vi "SPCC_Assignment_Simulation.vi"() -> ()   [LabVIEW 2023]
uses:
  e3bf969a-aac0-434e-a3ae-6fd923815a2a.vi
  48b219de-f1ff-457e-af6a-4fba154d072f.vi
  41e50873-912a-4f0f-ad4e-86c641a04fe7.vi
  6f4b4a78-1284-474b-8f97-6c78d8e6e227.vi
  13f19a0c-8ff0-4895-a446-3eb92896fe58.vi
  ebdab617-ba7c-440d-b82c-f0f3d50a62cd.vi
  86e3c8e6-2093-4571-a988-bd0a6019ca9d.vi
  4dc1e517-941c-447c-bbf6-cb1460c6f39a.vi
  a41b0926-84b4-47fe-bcd1-4c6ccf125de5.vi
  03f30388-958a-4886-846a-0cab3cf4eed9.vi
  04fb8fff-2e92-42f1-ae9c-eeda405f3134.vi
  4105182e-33e6-4150-80c3-b8c49d90c377.vi
panel:
  in  "btnStop":bool
  in  "A1":bool
  in  "A6":bool
  in  "A5":bool
  in  "A4":bool
  in  "A3":bool
  in  "A2":bool
  in  "B1":bool
  in  "B6":bool
  in  "B5":bool
  in  "B4":bool
  in  "B3":bool
  in  "B2":bool
  in  "T1":bool
  in  "T6":bool
  in  "T5":bool
  in  "T4":bool
  in  "T3":bool
  in  "T2":bool
  # "1"
  # "2"
  # "3"
  # "4"
  # "5"
  # "6"
  # "Zone"
  # "Alarm Switches"
  # "Bypass Switches"
  # "Tamper Switches"
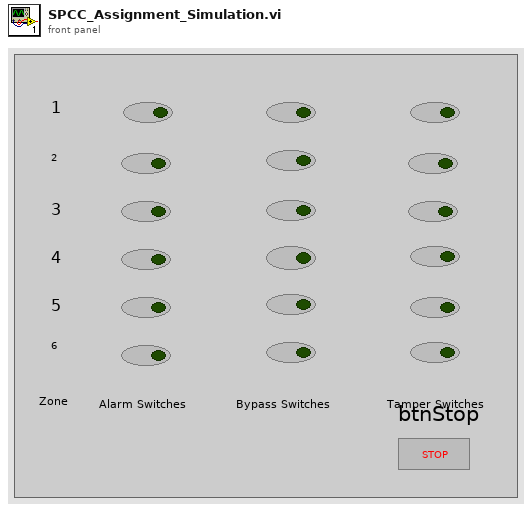
[diagram p1: front panel]
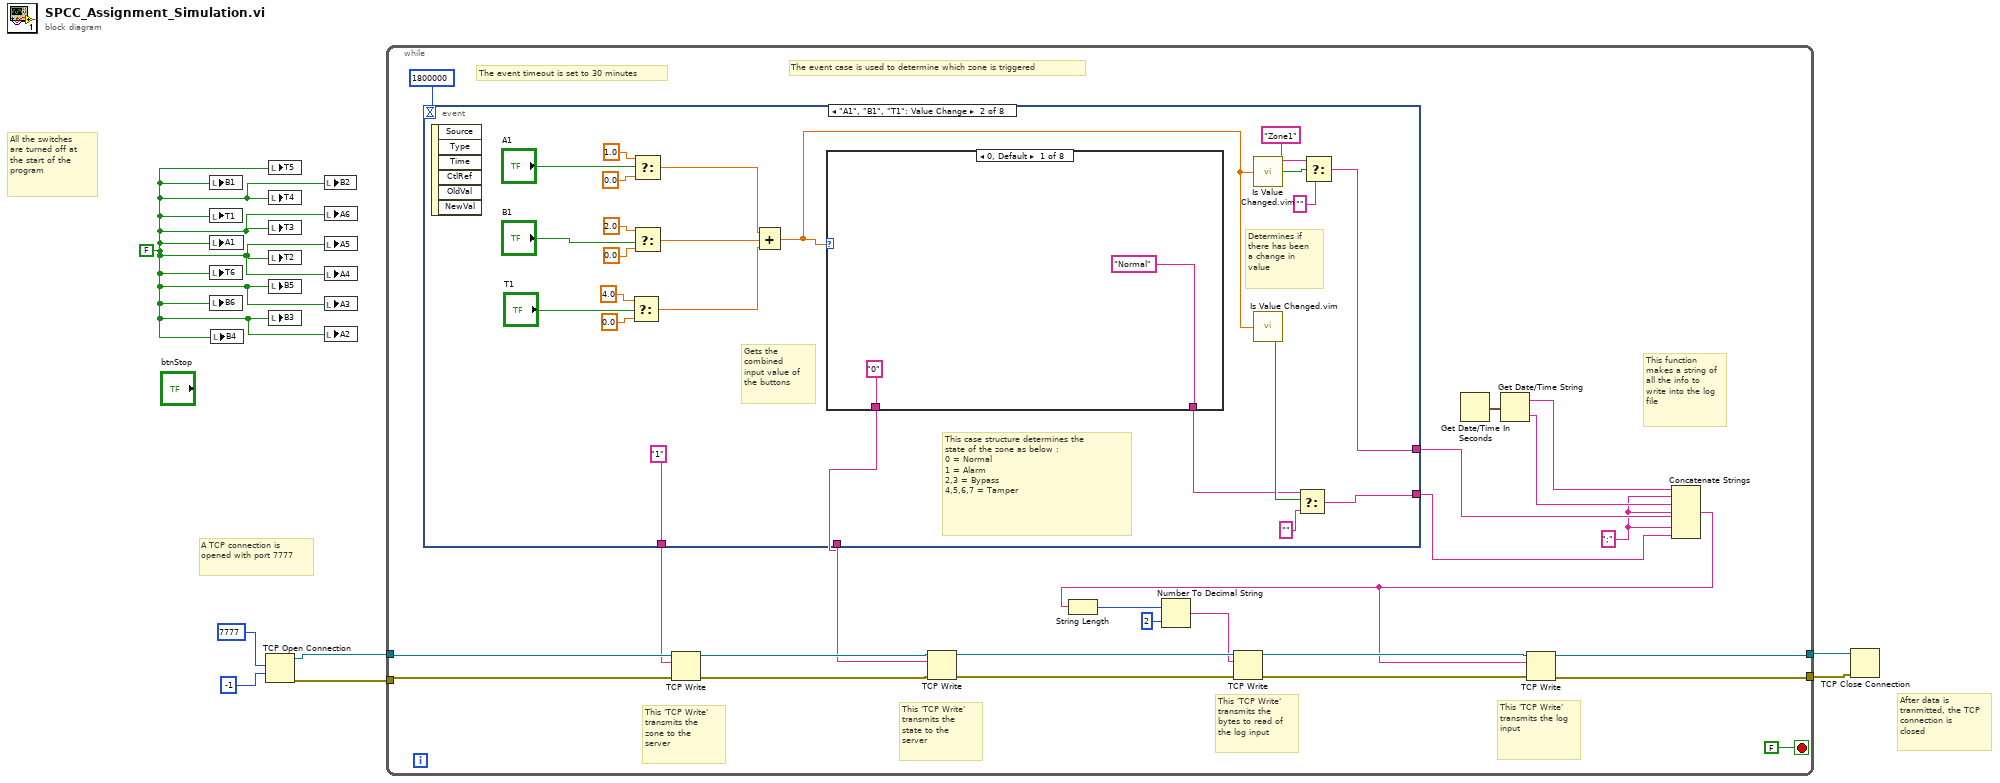
[diagram p0: block diagram]
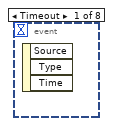
[diagram p2: hidden frame]
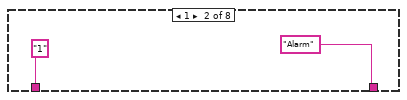
[diagram p3: hidden frame]
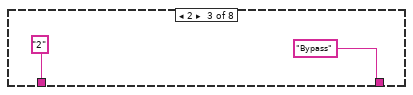
[diagram p4: hidden frame]
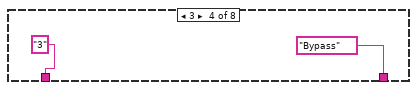
[diagram p5: hidden frame]
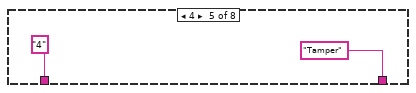
[diagram p6: hidden frame]
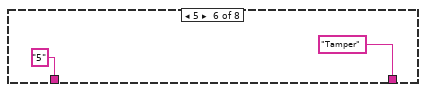
[diagram p7: hidden frame]
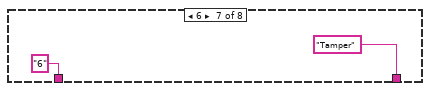
[diagram p8: hidden frame]
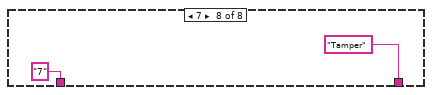
[diagram p9: hidden frame]
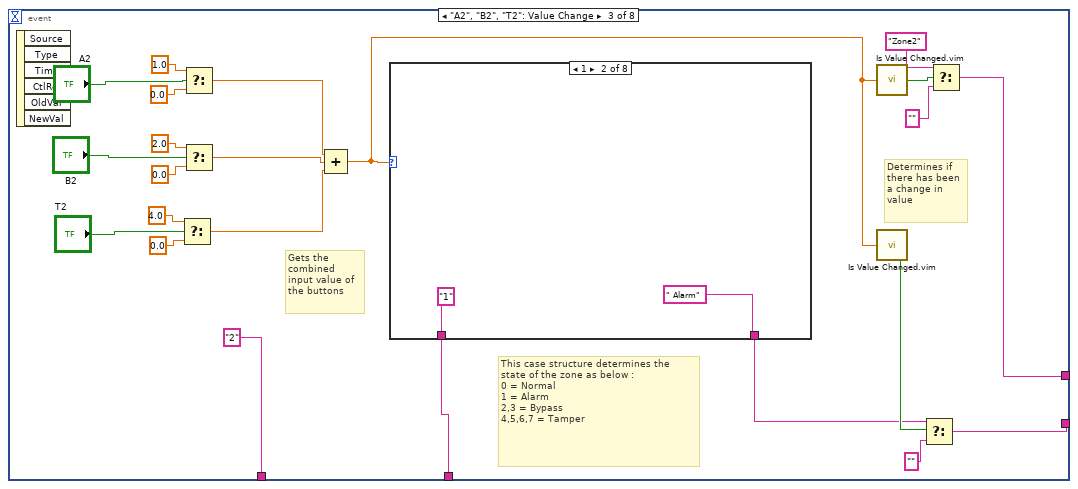
[diagram p10: hidden frame]
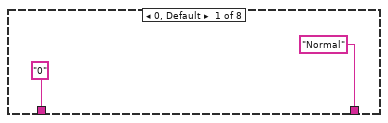
[diagram p11: hidden frame]
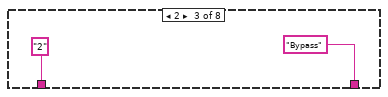
[diagram p12: hidden frame]
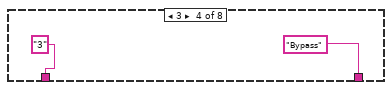
[diagram p13: hidden frame]
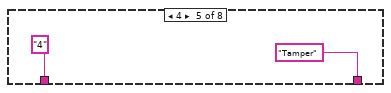
[diagram p14: hidden frame]
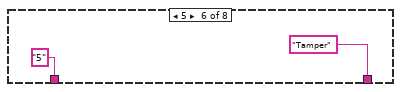
[diagram p15: hidden frame]
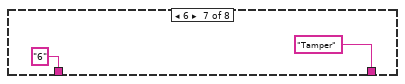
[diagram p16: hidden frame]
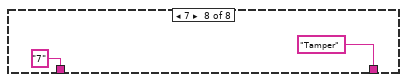
[diagram p17: hidden frame]
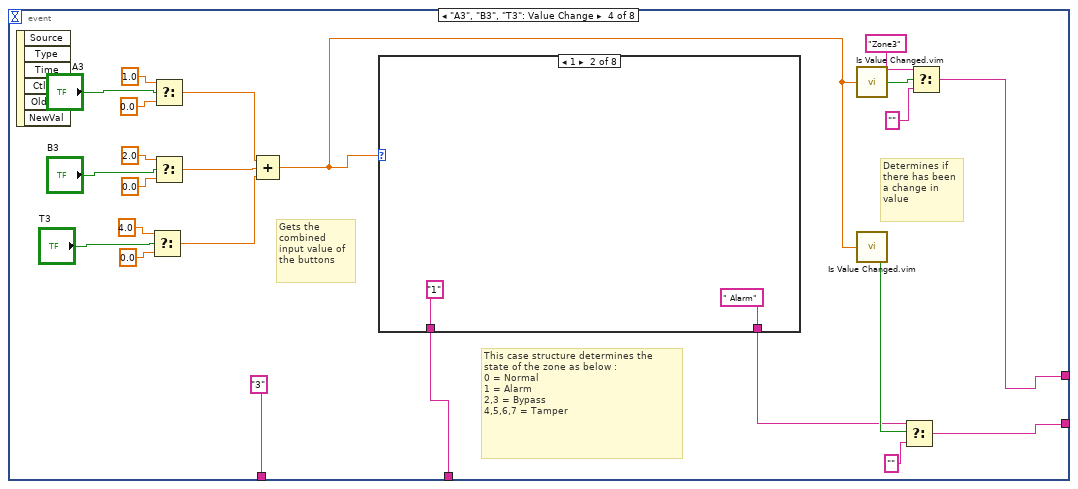
[diagram p18: hidden frame]
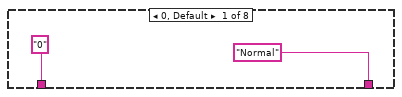
[diagram p19: hidden frame]
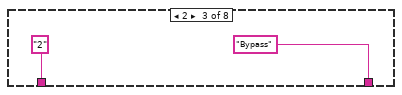
[diagram p20: hidden frame]
diagram:
  w7 = FALSE
  # "After data is tranmitted, the TCP connection is closed"
  # "A TCP connection is opened with port 7777"
  # "All the switches are turned off at the start of the program"
  n1 = local write "B1"(w7) -> ()
  n2 = local write "T1"(w7) -> ()
  n3 = local write "A1"(w7) -> ()
  n4 = local write "T6"(w7) -> ()
  n5 = local write "B6"(w7) -> ()
  n6 = local write "B4"(w7) -> ()
  n7 = TCP Open Connection(remote port or service name=u16 7777, timeout ms (60000)=-1) -> (connection ID=w3:refnum<k5>, error out=w4:errorcluster)  [unwired: 3 in]
  n8 = local write "T5"(w7) -> ()
  n9 = local write "T4"(w7) -> ()
  n10 = local write "T3"(w7) -> ()
  n11 = local write "T2"(w7) -> ()
  n12 = local write "B5"(w7) -> ()
  n13 = local write "B3"(w7) -> ()
  n14 = local write "B2"(w7) -> ()
  n15 = local write "A6"(w7) -> ()
  n16 = local write "A5"(w7) -> ()
  n17 = local write "A4"(w7) -> ()
  n18 = local write "A3"(w7) -> ()
  n19 = local write "A2"(w7) -> ()
  n20 = while {
    tunnel: [w21] -> w6
    tunnel: [w22] -> w5
    tunnel: w4 -> [w31]
    tunnel: w3 -> [w30]
    stop <- FALSE stop-if-true
    w18 = ";" ("delimiter (\\t)")
    # "This function makes a string of all the info to write into the log file"
    # "This 'TCP Write' transmits the log input"
    # "This 'TCP Write' transmits the bytes to read of the log input"
    # "This 'TCP Write' transmits the state to the server"
    # "This 'TCP Write' transmits the zone to the server"
    # "The event timeout is set to 30 minutes"
    # "The event case is used to determine which zone is triggered"
    n21 = event shown="[1] \"A1\", \"B1\", \"T1\": Value Change" {
      selector: _ -> [_ _ _ _ _ _ _ _]
      dyn-events: _ -> [_ _ _ _ _ _ _ _]
      timeout: 1800000 -> [_ _ _ _ _ _ _ _]
      tunnel: [_ "1" "2" ("data in") "3" "4" "5" "6" _] -> w27
      tunnel: [_ w45 w83 w123 w161 w201 w239 _] -> w26
      tunnel: [_ w42 w74 w114 w153 w192 w231 _] -> w17
      tunnel: [_ w38 w75 w115 w154 w193 w232 _] -> w19
      event Timeout {
        n22 = event-data() -> ()  [unwired: 1 in, 3 out]
      }
      event "A1", "B1", "T1": Value Change {
        # "Gets the combined input value of the buttons"
        # "Determines if there has been a change in value"
        # "This case structure determines the state of the zone as below :\n0 = Normal\n1 = Alarm\n2,3 = Bypass\n4,5,6,7 = Tamper"
        n23 = event-data() -> ()  [unwired: 1 in, 6 out]
        n24 = Select(t=4.0, s="T1", f=0.0) -> (s? t:f=w52:dbl)
        n25 = Select(t=1.0, s="A1", f=0.0) -> (s? t:f=w54:dbl)
        n26 = Select(t=2.0, s="B1", f=0.0) -> (s? t:f=w53:dbl)
        n27 = Compound Arithmetic op=ADD(w54, w53, w52) -> (w41:dbl)
        n28 = case shown="0, Default" w41 {
          tunnel: ["0" "1" "2" "3" "4" "5" "6" "7"] -> w45
          tunnel: ["Normal" "Alarm" "Bypass" "Bypass" "Tamper" "Tamper" "Tamper" "Tamper"] -> w37
          frame 0, Default {
          }
          frame 1 {
          }
          frame 2 {
          }
          frame 3 {
          }
          frame 4 {
          }
          frame 5 {
          }
          frame 6 {
          }
          frame 7 {
          }
        }
        n29 = call "Is Value Changed.vim"("value"=w41) -> ("changed or first call?"=w40:bool)
        n30 = call "Is Value Changed.vim"("value"=w41) -> ("changed or first call?"=w43:bool)
        n31 = Select(t=w37, s=w43, f="") -> (s? t:f=w42:string)
        n32 = Select(t="Zone1", s=w40, f="") -> (s? t:f=w38:string)
      }
      event "A2", "B2", "T2": Value Change {
        # "Determines if there has been a change in value"
        # "Gets the combined input value of the buttons"
        # "This case structure determines the state of the zone as below :\n0 = Normal\n1 = Alarm\n2,3 = Bypass\n4,5,6,7 = Tamper"
        n33 = event-data() -> ()  [unwired: 1 in, 6 out]
        n34 = Select(t=4.0, s="T2", f=0.0) -> (s? t:f=w91:dbl)
        n35 = Select(t=1.0, s="A2", f=0.0) -> (s? t:f=w93:dbl)
        n36 = Select(t=2.0, s="B2", f=0.0) -> (s? t:f=w92:dbl)
        n37 = Compound Arithmetic op=ADD(w93, w92, w91) -> (w77:dbl)
        n38 = case shown="1" w77 {
          tunnel: ["0" "1" "2" "3" "4" "5" "6" "7"] -> w83
          tunnel: ["Normal" " Alarm" "Bypass" "Bypass" "Tamper" "Tamper" "Tamper" "Tamper"] -> w76
          frame 0, Default {
          }
          frame 1 {
          }
          frame 2 {
          }
          frame 3 {
          }
          frame 4 {
          }
          frame 5 {
          }
          frame 6 {
          }
          frame 7 {
          }
        }
        n39 = call "Is Value Changed.vim"("value"=w77) -> ("changed or first call?"=w81:bool)
        n40 = call "Is Value Changed.vim"("value"=w77) -> ("changed or first call?"=w82:bool)
        n41 = Select(t=w76, s=w82, f="") -> (s? t:f=w74:string)
        n42 = Select(t="Zone2", s=w81, f="") -> (s? t:f=w75:string)
      }
      event "A3", "B3", "T3": Value Change {
        # "Determines if there has been a change in value"
        # "Gets the combined input value of the buttons"
        # "This case structure determines the state of the zone as below :\n0 = Normal\n1 = Alarm\n2,3 = Bypass\n4,5,6,7 = Tamper"
        n43 = event-data() -> ()  [unwired: 1 in, 6 out]
        n44 = Select(t=4.0, s="T3", f=0.0) -> (s? t:f=w130:dbl)
        n45 = Select(t=1.0, s="A3", f=0.0) -> (s? t:f=w132:dbl)
        n46 = Select(t=2.0, s="B3", f=0.0) -> (s? t:f=w131:dbl)
        n47 = Compound Arithmetic op=ADD(w132, w131, w130) -> (w116:dbl)
        n48 = case shown="1" w116 {
          tunnel: ["0" "1" "2" "3" "4" "5" "6" "7"] -> w123
          tunnel: ["Normal" " Alarm" "Bypass" "Bypass" "Tamper" "Tamper" "Tamper" "Tamper"] -> w113
          frame 0, Default {
          }
          frame 1 {
          }
          frame 2 {
          }
          frame 3 {
          }
          frame 4 {
          }
          frame 5 {
          }
          frame 6 {
          }
          frame 7 {
          }
        }
        n49 = call "Is Value Changed.vim"("value"=w116) -> ("changed or first call?"=w120:bool)
        n50 = call "Is Value Changed.vim"("value"=w116) -> ("changed or first call?"=w121:bool)
        n51 = Select(t=w113, s=w121, f="") -> (s? t:f=w114:string)
        n52 = Select(t="Zone3", s=w120, f="") -> (s? t:f=w115:string)
      }
      event "A4", "B4", "T4": Value Change {
        # "Determines if there has been a change in value"
        # "Gets the combined input value of the buttons"
        # "This case structure determines the state of the zone as below :\n0 = Normal\n1 = Alarm\n2,3 = Bypass\n4,5,6,7 = Tamper"
        n53 = event-data() -> ()  [unwired: 1 in, 6 out]
        n54 = Select(t=4.0, s="T4", f=0.0) -> (s? t:f=w169:dbl)
        n55 = Select(t=1.0, s="A4", f=0.0) -> (s? t:f=w171:dbl)
        n56 = Select(t=2.0, s="B4", f=0.0) -> (s? t:f=w170:dbl)
        n57 = Compound Arithmetic op=ADD(w171, w170, w169) -> (w155:dbl)
        n58 = case shown="1" w155 {
          tunnel: ["0" "1" "2" "3" "4" "5" "6" "7"] -> w161
          tunnel: ["Normal" " Alarm" "Bypass" "Bypass" "Tamper" "Tamper" "Tamper" "Tamper"] -> w152
          frame 0, Default {
          }
          frame 1 {
          }
          frame 2 {
          }
          frame 3 {
          }
          frame 4 {
          }
          frame 5 {
          }
          frame 6 {
          }
          frame 7 {
          }
        }
        n59 = call "Is Value Changed.vim"("value"=w155) -> ("changed or first call?"=w159:bool)
        n60 = call "Is Value Changed.vim"("value"=w155) -> ("changed or first call?"=w160:bool)
        n61 = Select(t=w152, s=w160, f="") -> (s? t:f=w153:string)
        n62 = Select(t="Zone4", s=w159, f="") -> (s? t:f=w154:string)
      }
      event "A5", "B5", "T5": Value Change {
        # "Determines if there has been a change in value"
        # "Gets the combined input value of the buttons"
        # "This case structure determines the state of the zone as below :\n0 = Normal\n1 = Alarm\n2,3 = Bypass\n4,5,6,7 = Tamper"
        n63 = event-data() -> ()  [unwired: 1 in, 6 out]
        n64 = Select(t=4.0, s="T5", f=0.0) -> (s? t:f=w208:dbl)
        n65 = Select(t=1.0, s="A5", f=0.0) -> (s? t:f=w210:dbl)
        n66 = Select(t=2.0, s="B5", f=0.0) -> (s? t:f=w209:dbl)
        n67 = Compound Arithmetic op=ADD(w210, w209, w208) -> (w194:dbl)
        n68 = case shown="0, Default" w194 {
          tunnel: ["0" "1" "2" "3" "4" "5" "6" "7"] -> w201
          tunnel: ["Normal" " Alarm" "Bypass" "Bypass" "Tamper" "Tamper" "Tamper" "Tamper"] -> w191
          frame 0, Default {
          }
          frame 1 {
          }
          frame 2 {
          }
          frame 3 {
          }
          frame 4 {
          }
          frame 5 {
          }
          frame 6 {
          }
          frame 7 {
          }
        }
        n69 = call "Is Value Changed.vim"("value"=w194) -> ("changed or first call?"=w198:bool)
        n70 = call "Is Value Changed.vim"("value"=w194) -> ("changed or first call?"=w199:bool)
        n71 = Select(t=w191, s=w199, f="") -> (s? t:f=w192:string)
        n72 = Select(t="Zone5", s=w198, f="") -> (s? t:f=w193:string)
      }
      event "A6", "B6", "T6": Value Change {
        # "Determines if there has been a change in value"
        # "Gets the combined input value of the buttons"
        # "This case structure determines the state of the zone as below :\n0 = Normal\n1 = Alarm\n2,3 = Bypass\n4,5,6,7 = Tamper"
        n73 = event-data() -> ()  [unwired: 1 in, 6 out]
        n74 = Select(t=4.0, s="T6", f=0.0) -> (s? t:f=w247:dbl)
        n75 = Select(t=2.0, s="B6", f=0.0) -> (s? t:f=w248:dbl)
        n76 = Select(t=1.0, s="A6", f=0.0) -> (s? t:f=w249:dbl)
        n77 = Compound Arithmetic op=ADD(w249, w248, w247) -> (w233:dbl)
        n78 = case shown="1" w233 {
          tunnel: ["0" "1" "2" "3" "4" "5" "6" "7"] -> w239
          tunnel: ["Normal" " Alarm" "Bypass" "Bypass" "Tamper" "Tamper" "Tamper" "Tamper"] -> w230
          frame 0, Default {
          }
          frame 1 {
          }
          frame 2 {
          }
          frame 3 {
          }
          frame 4 {
          }
          frame 5 {
          }
          frame 6 {
          }
          frame 7 {
          }
        }
        n79 = call "Is Value Changed.vim"("value"=w233) -> ("changed or first call?"=w237:bool)
        n80 = call "Is Value Changed.vim"("value"=w233) -> ("changed or first call?"=w238:bool)
        n81 = Select(t=w230, s=w238, f="") -> (s? t:f=w231:string)
        n82 = Select(t="Zone6", s=w237, f="") -> (s? t:f=w232:string)
      }
      event "btnStop": Mouse Up {
        # "This case stops the program when the 'btnStop' is clicked"
        n83 = event-data() -> ()  [unwired: 1 in, 8 out]
        n84 = Stop(stop? (T)=TRUE) -> ()
      }
    }
    n85 = TCP Write(connection ID=w30, data in=w27, error in (no error)=w31) -> (connection ID out=w28:refnum<k5>, error out=w29:errorcluster)  [unwired: 1 in, 1 out]
    n86 = TCP Write(connection ID=w28, data in=w26, error in (no error)=w29) -> (connection ID out=w14:refnum<k5>, error out=w12:errorcluster)  [unwired: 1 in, 1 out]
    n87 = Get Date/Time In Seconds() -> (seconds since 1Jan1904=w24:timestamp)
    n88 = Get Date/Time String(seconds (now)=w24) -> (date string=w23:string, time string=w20:string)  [unwired: 2 in]
    n89 = Concatenate Strings "Concatenate Strings"(w23, w18, w20, w18, w19, w18, w17) -> (w9:string)
    n90 = String Length(string=w9) -> (length=w16:i32)
    n91 = Number To Decimal String(number=w16, width (-)=i16 2) -> (decimal integer string=w10:string)
    n92 = TCP Write(connection ID=w14, data in=w10, error in (no error)=w12) -> (connection ID out=w13:refnum<k5>, error out=w11:errorcluster)  [unwired: 1 in, 1 out]
    n93 = TCP Write(connection ID=w13, data in=w9, error in (no error)=w11) -> (connection ID out=w22:refnum<k5>, error out=w21:errorcluster)  [unwired: 1 in, 1 out]
  }
  n94 = TCP Close Connection(connection ID=w5, error in (no error)=w6) -> ()  [unwired: 1 in, 2 out]
